vi "random_between.vi"(4 "b":dbl, 5 "a":dbl) -> (1 "Random":dbl)   [LabVIEW 2016]
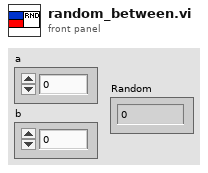
[diagram p1: front panel]
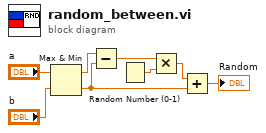
[diagram p0: block diagram]
diagram:
  n1 = Max & Min(x="a", y="b") -> (max(x,y)=w2:dbl, min(x,y)=w1:dbl)
  n2 = Subtract(x=w2, y=w1) -> (x-y=w8:dbl)
  n3 = Random Number (0-1)() -> (number: 0 to 1=w7:dbl)
  n4 = Multiply(x=w8, y=w7) -> (x*y=w6:dbl)
  n5 = Add(x=w6, y=w1) -> (x+y=→"Random":dbl)
